vi "Read CH 1 Max Outputs.vi"(8 "error in (no error)":errorcluster, 11 "2230G in":refnum<class "2230G.lvclass">) -> (0 "error out":errorcluster, 2 "CH 1 Max Outputs":cluster{"Voltage (V)":dbl, "Current (A)":dbl}={"Voltage (V)"=30.0, "Current (A)"=3.0}, 3 "2230G out":refnum<class "2230G.lvclass">)   [LabVIEW 2018, in "2230G.lvlib" / "2230G.lvclass"]
uses:
  2230G.lvclass
  2230G.lvclass/2230G.ctl
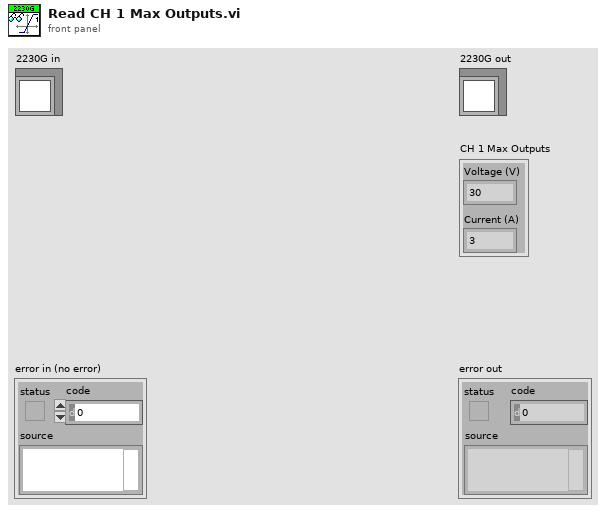
[diagram p1: front panel]
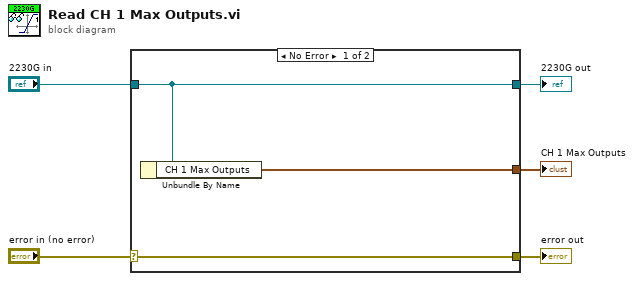
[diagram p0: block diagram]
diagram:
  n1 = case shown="No Error" "error in (no error)" {
    selector: "error in (no error)" -> [w8 w9]
    tunnel: [w8 w9] -> w4
    tunnel: [w7 w10] -> w2
    tunnel: "2230G in" -> [w7 w10]
    tunnel: [w6 _] -> w1
    frame No Error {
      n2 = Unbundle By Name(w7) -> ("CH 1 Max Outputs"=w6:cluster{"Voltage (V)":dbl, "Current (A)":dbl})
    }
    frame Error {
    }
  }
  "error out" <- w4
  "2230G out" <- w2
  "CH 1 Max Outputs" <- w1
